vi "MT Apply Flat Fading Profile.vi"(0 "input complex waveform":T1={"t0"=0.0, "dt"=1.0, "Y"=[]} {"Y" format="%.3f"; "dt" format="%^.2e"; "t0" format="%.4f"}, 5 "fading profile":cdb[](array[numeric]) format="%.2f", 11 "error in (no error)":errorcluster, 13 "reset? (T)":bool=TRUE) -> (4 "output complex waveform":T1 {"Y" format="%.3f"; "dt" format="%^.2e"; "t0" format="%.4f"}, 15 "error out":errorcluster)   [LabVIEW 2020, in "niDMT.lvlib"]
doc: "Applies a flat fading profile to the <B>input complex waveform</B>."
uses:
  <vilib>/addons/Modulation/niDMT.lvlib
  <vilib>/addons/Modulation/Analog/controls/Complex Data Waveform.ctl
  <vilib>/Analysis/baseanly.llb/Mean (DBL).vi
  <vilib>/Analysis/baseanly.llb/Mean (CDB).vi
  <vilib>/addons/Modulation/niAMT.lvlib
  <vilib>/Analysis/NI_AALBase.lvlib
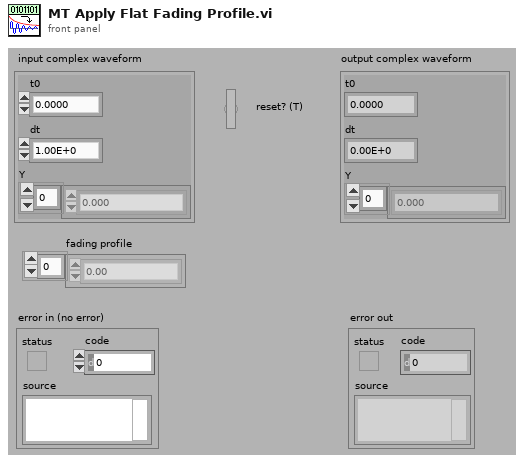
[diagram p1: front panel]
types:
  T1 = typedef "niAMT.lvlib/Complex Data Waveform.ctl" = cluster{"t0":dbl, "dt":dbl, "Y":cdb[]}
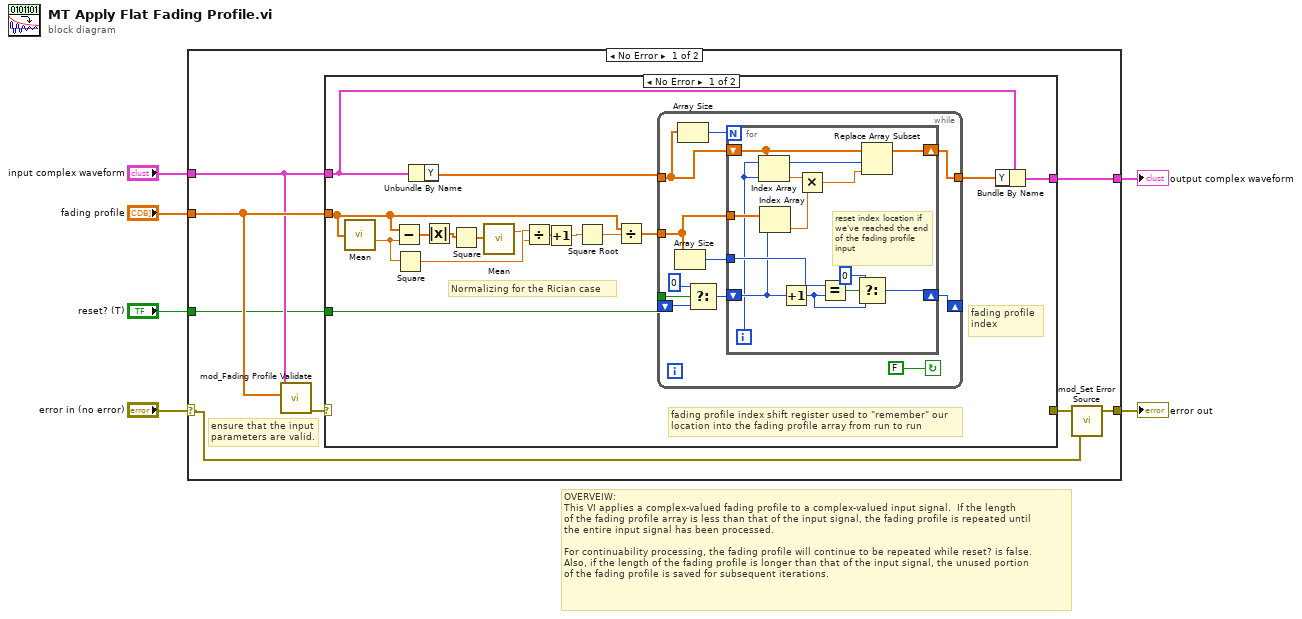
[diagram p0: block diagram]
diagram:
  # "OVERVEIW:\nThis VI applies a complex-valued fading profile to a complex-valued input signal.  If the length\nof the fading profile array is less than that of the input signal, the fading profile is repeated until\nthe entire input signal has been processed.\n\nFor continuability processing, the fading profile will continue to be repeated while reset? is false.\nAlso, if the length of the fading profile is longer than that of the input signal, the unused portion\nof the fading profile is saved for subsequent iterations."
  n1 = case shown="No Error" "error in (no error)" {
    selector: "error in (no error)" -> [w7 w56]
    tunnel: "input complex waveform" -> [w12 _]
    tunnel: "fading profile" -> [w13 _]
    tunnel: "reset? (T)" -> [w11 _]
    tunnel: [w10 _] -> w2
    tunnel: [w9 w56] -> w1
    frame No Error {
      # "ensure that the input parameters are valid."
      n2 = call <vilib>:"mod_Fading Profile Validate.vi"("Fading Profile"=w13, "Input Complex Waveform"=w12) -> ("error out"=w14:errorcluster)  [unwired: 9 out]
      n3 = case shown="No Error" w14 {
        selector: w14 -> [_ w55]
        tunnel: w13 -> [w17 _]
        tunnel: w12 -> [w27 _]
        tunnel: w11 -> [w29 _]
        tunnel: [w26 _] -> w10
        tunnel: [_ w55] -> w8
        frame No Error {
          # "Normalizing for the Rician case"
          # "fading profile\nindex"
          # "fading profile index shift register used to \"remember\" our location into the fading profile array from run to run"
          n4 = call-poly <vilib>:"Mean.vi"("X"=w17) -> ("mean"=w22:cdb)  [unwired: 1 out]
          n5 = Subtract(x=w17, y=w22) -> (x-y=w25:cdb[])
          n6 = Square(x=w22) -> (x^2=w21:cdb)
          n7 = Unbundle By Name(w27) -> ("Y"=w30:cdb[])
          n8 = Absolute Value(x=w25) -> (abs(x)=w24:dbl[])
          n9 = Square(x=w24) -> (x^2=w23:dbl[])
          n10 = call-poly <vilib>:"Mean.vi"("X"=w23) -> ("mean"=w20:dbl)  [unwired: 1 out]
          n11 = Divide(x=w21, y=w20) -> (x/y=w19:cdb)
          n12 = Increment(x=w19) -> (x+1=w18:cdb)
          n13 = Square Root(x=w18) -> (sqrt(x)=w15:cdb)
          n14 = Divide(x=w17, y=w15) -> (x/y=w16:cdb[])
          n15 = while {
            shift-right: [w36] -> _
            shift-left: _ -> [w41]
            tunnel: w30 -> [w33]
            tunnel: w29 -> [w39]
            tunnel: w16 -> [w37]
            tunnel: [w31] -> w28
            stop <- FALSE continue-if-true
            n16 = Array Size(array=w37) -> (size(s)=w34:i32)
            n17 = Array Size(array=w33) -> (size(s)=w32:i32)
            n18 = Select(t=0, s=w39, f=w41) -> (s? t:f=w40:i32)
            n19 = for {
              N: w32 -> [_]
              shift-right: [w50] -> w36
              shift-left: w40 -> [w48]
              tunnel: w37 -> [w49]
              tunnel: w34 -> [w53]
              shift-right: [w43] -> w31
              shift-left: w33 -> [w42]
              i -> [w46]
              # "reset index location if we've reached the end of the fading profile input"
              n20 = Index Array(array=w42, index=w46) -> (element=w44:cdb)
              n21 = Index Array(array=w49, index=w48) -> (element=w47:cdb)
              n22 = Increment(x=w48) -> (x+1=w51:i32)
              n23 = Multiply(x=w44, y=w47) -> (x*y=w45:cdb)
              n24 = Equal?(x=w53, y=w51) -> (x = y?=w54:bool)
              n25 = Select(t=0, s=w54, f=w51) -> (s? t:f=w50:i32)
              n26 = Replace Array Subset(array=w42, new element=w45, index=w46) -> (w43:cdb[])
            }
          }
          n27 = Bundle By Name(cluster=w27, "Y"=w28) -> (w26:T1)
        }
        frame Error {
        }
      }
      n28 = call <vilib>:"mod_Set Error Source.vi"("initial error in (no error)"=w7, "final error in (no error)"=w8) -> ("error out"=w9:errorcluster)  [unwired: 1 in, 2 out]
    }
    frame Error {
    }
  }
  "error out" <- w1
  "output complex waveform" <- w2
